vi "oa_Check Param Changes.vi"(7 "Reset?":bool, 8 "param4":variant, 9 "param3":variant, 10 "param2":variant, 11 "param1":variant) -> (5 "Reset out":bool)   [LabVIEW 2017]
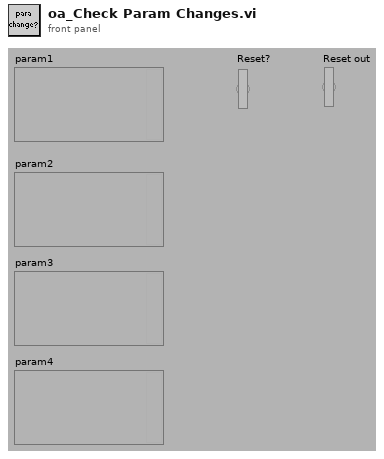
[diagram p1: front panel]
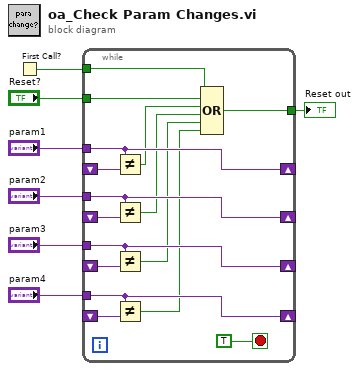
[diagram p0: block diagram]
diagram:
  n1 = First Call?() -> (First Call?: T/F=w1:bool)
  n2 = while {
    shift-right: [w21] -> _
    shift-left: _ -> [w22]
    tunnel: "param1" -> [w21]
    shift-right: [w20] -> _
    shift-left: _ -> [w19]
    tunnel: "param2" -> [w20]
    shift-right: [w17] -> _
    shift-left: _ -> [w18]
    tunnel: "param3" -> [w17]
    shift-right: [w16] -> _
    shift-left: _ -> [w15]
    tunnel: "param4" -> [w16]
    tunnel: "Reset?" -> [w14]
    tunnel: [w9] -> w2
    tunnel: w1 -> [w8]
    stop <- TRUE stop-if-true
    n3 = Not Equal?(x=w21, y=w22) -> (x != y?=w13:bool)
    n4 = Not Equal?(x=w20, y=w19) -> (x != y?=w12:bool)
    n5 = Not Equal?(x=w17, y=w18) -> (x != y?=w11:bool)
    n6 = Not Equal?(x=w16, y=w15) -> (x != y?=w10:bool)
    n7 = Compound Arithmetic op=OR(w8, w14, w13, w12, w11, w10) -> (w9:bool)
  }
  "Reset out" <- w2
